vi "S2C_VLFT10_Proc_StringToDateTime.vi"(8 "Error In":errorcluster, 10 "Format String":string, 11 "DateTime String":string) -> (0 "Error Out":errorcluster, 3 "TimeStamp":timestamp)   [LabVIEW 2015]
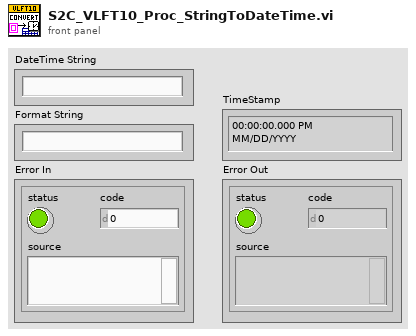
[diagram p1: front panel]
types:
  T1 = cluster{"second":i32, "minute":i32, "hour":i32, "day of month":i32, "month":i32, "year":i32, "day of week":i32, "day of year":i32, "is DST":i32}
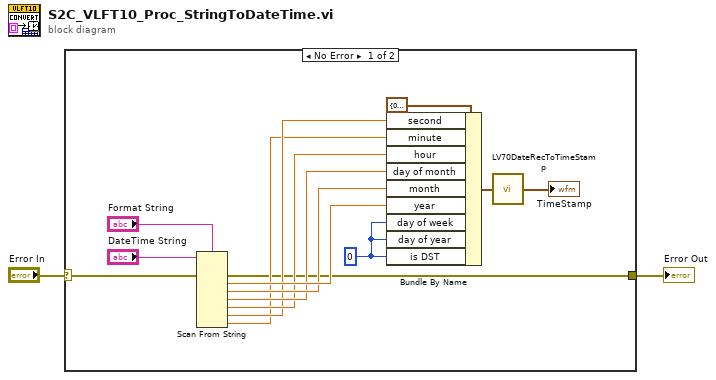
[diagram p0: block diagram]
diagram:
  n1 = case shown="No Error" "Error In" {
    selector: "Error In" -> [w3 w17]
    tunnel: [w4 w17] -> w2
    frame No Error {
      w15 = 0
      n2 = Scan From String(format string="Format String", input string="DateTime String", error in=w3) -> (error out=w4:errorcluster, output 1=w14:dbl, output 2=w13:dbl, output 3=w12:dbl, output 4=w11:dbl, output 5=w10:dbl, output 6=w9:dbl)  [unwired: 7 in, 2 out]
      n3 = Bundle By Name(cluster=T1 {"second"=0, "minute"=0, "hour"=0, "day of month"=0, "month"=0, "year"=0, "day of week"=0, "day of year"=0, "is DST"=0} ("date time rec"), "second"=w10, "minute"=w9, "hour"=w11, "day of month"=w12, "month"=w13, "year"=w14, "day of week"=w15, "day of year"=w15, "is DST"=w15) -> (w8:T1)
      n4 = call <vilib>:"LV70DateRecToTimeStamp.vi"("date time rec"=w8) -> ("Time Stamp"=→"TimeStamp":timestamp)
    }
    frame Error {
    }
  }
  "Error Out" <- w2
